vi "3P_filestruct.vi"(6 "Batteryname":string, 8 "For loop i":i32, 9 "In for loop":bool, 11 "Starting Cycle":i32) -> (0 "DischargeWaitPath":path, 1 "DischargeCyclePath":path, 2 "ChargeWaitPath":path, 3 "ChargeCyclePath":path, 5 "Cycle Index":i32)   [LabVIEW 2020]
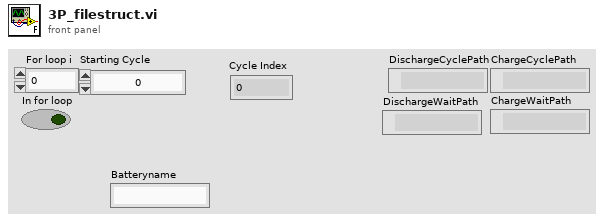
[diagram p1: front panel]
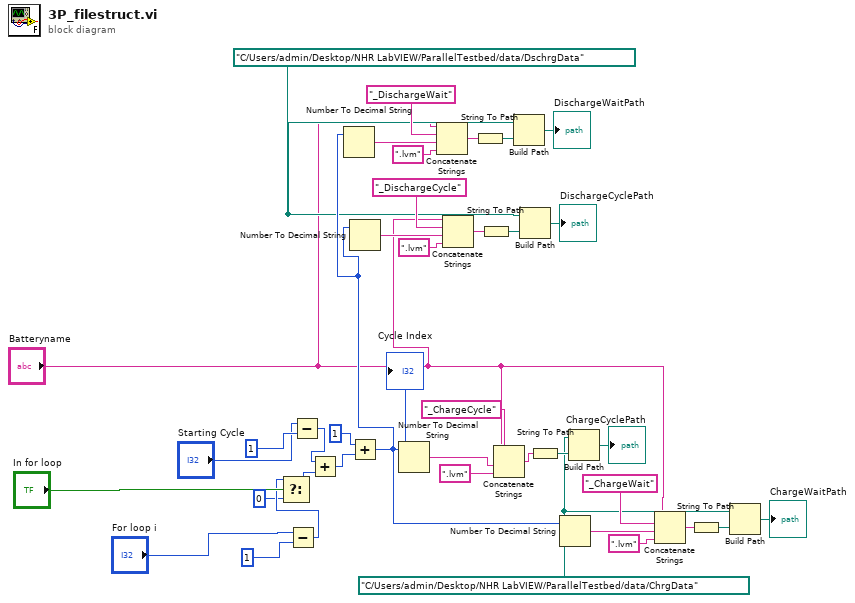
[diagram p0: block diagram]
diagram:
  w18 = path "C:/Users/admin/Desktop/NHR LabVIEW/ParallelTestbed/data/ChrgData" ("base path")
  w19 = path "C:/Users/admin/Desktop/NHR LabVIEW/ParallelTestbed/data/DschrgData" ("base path")
  n1 = Subtract(x="For loop i", y=1) -> (x-y=w10:i32)
  n2 = Select(t=w10, s="In for loop", f=0) -> (s? t:f=w8:i32)
  n3 = Subtract(x="Starting Cycle", y=1) -> (x-y=w5:i32)
  n4 = Add(x=w5, y=w8) -> (x+y=w20:i32)
  n5 = Add(x=1, y=w20) -> (x+y=w21:i32)
  "Cycle Index" <- w21
  n6 = Number To Decimal String(number=w21) -> (decimal integer string=w28:string)  [unwired: 1 in]
  n7 = Number To Decimal String(number=w21) -> (decimal integer string=w33:string)  [unwired: 1 in]
  n8 = Number To Decimal String(number=w21) -> (decimal integer string=w3:string)  [unwired: 1 in]
  n9 = Concatenate Strings("Batteryname", "_DischargeWait", w28, ".lvm") -> (w29:string)
  n10 = Concatenate Strings("Batteryname", "_DischargeCycle", w33, ".lvm") -> (w34:string)
  n11 = String To Path(string=w29) -> (path=w30:path)
  n12 = String To Path(string=w34) -> (path=w35:path)
  n13 = Concatenate Strings("Batteryname", "_ChargeCycle", w3, ".lvm") -> (w37:string)
  n14 = Build Path(base path=w19, name or relative path=w30) -> (appended path=→"DischargeWaitPath":path)
  n15 = Build Path(base path=w19, name or relative path=w35) -> (appended path=→"DischargeCyclePath":path)
  n16 = String To Path(string=w37) -> (path=w38:path)
  n17 = Number To Decimal String(number=w21) -> (decimal integer string=w23:string)  [unwired: 1 in]
  n18 = Build Path(base path=w18, name or relative path=w38) -> (appended path=→"ChargeCyclePath":path)
  n19 = Concatenate Strings("Batteryname", "_ChargeWait", w23, ".lvm") -> (w24:string)
  n20 = String To Path(string=w24) -> (path=w25:path)
  n21 = Build Path(base path=w18, name or relative path=w25) -> (appended path=→"ChargeWaitPath":path)
